vi "Teleop.vi"(10 "Match Info":T1={"Autonomous Elapsed Seconds"=0.0, "TeleOp Elapsed Seconds"=0.0, "Disabled Elapsed Seconds"=0.0, "Visited Autonomous"=FALSE, "Visited TeleOp"=FALSE, "Visited Disabled"=FALSE, "Autonomous Settings"={"Autonomous Style"=enum."Independent", "VI Refnum"=refnum}}, 11 "Call Context":T2) -> ()   [LabVIEW 2017]
doc: "This VI is called for each TeleOp packet received from the DS where the robot is not disabled. It is often used to read from the joysticks and update I/O or to update setpoints for timed control loops. It should complete and return within 20 milliseconds or it may miss DS packets."
uses:
  <vilib>/Rock Robotics/WPI/DriverStation/WPI_DriverStationDerivedRobotMode.ctl
  <vilib>/Rock Robotics/WPI/DriverStation/WPI_DriverStationMatch Info.ctl
  <vilib>/Rock Robotics/WPI/Utilities/WPI_GetSetVariantRefNum.vi
  <vilib>/Rock Robotics/Network Tables/NT Write Boolean Array.vi
  <vilib>/Rock Robotics/Network Tables/NT Write Numeric Array.vi
  <vilib>/Rock Robotics/Network Tables/NT Read Boolean.vi
  <vilib>/Rock Robotics/Network Tables/NT Read Number.vi
panel:
  in  "Lift Select":dbl
  out "Sample Slider 0":dbl(slide) scale=0.0..5.0
  out "Sample Boolean 1":bool
  out "Sample Boolean 0":bool
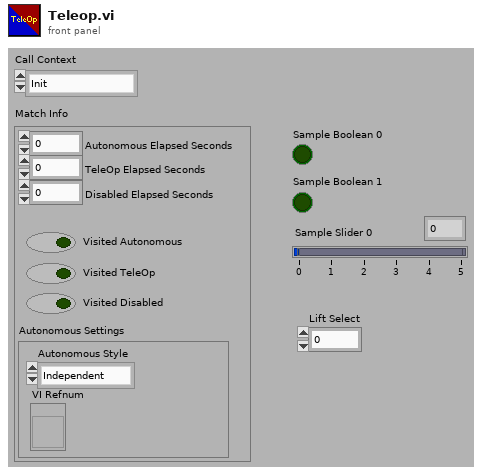
[diagram p1: front panel]
types:
  T1 = typedef "WPI_DriverStationMatch Info.ctl" = cluster{"Autonomous Elapsed Seconds":dbl, "TeleOp Elapsed Seconds":dbl, "Disabled Elapsed Seconds":dbl, "Visited Autonomous":bool, "Visited TeleOp":bool, "Visited Disabled":bool, "Autonomous Settings":cluster{"Autonomous Style":enum16{"Iterative", "Independent"}, "VI Refnum":refnum<vi>}}
  T2 = typedef "WPI_DriverStationDerivedRobotMode.ctl" = enum16{"Init", "Execute", "Stop"}
  T3 = typedef "WPI_JoystickDevRef.ctl" = cluster{"Device":T4}
  T4 = typedef "WPI_JoystickDeviceEnum.ctl" = enum16{"USB 0", "USB 1", "USB 2", "USB 3", "USB 4", "USB 5"}
  T5 = typedef "WPI_MotorControlDeviceRef.ctl" = cluster{"DeviceStatus":errorcluster, "Type":T6, "PWM":cluster{"PWM Channel":T7, "DeadBand":T8}, "CAN":cluster{"Device Number":u8, "SetOutput VI Ref":variant, "GetOutput VI Ref":variant, "Enable VI Ref":variant, "Disable VI Ref":variant, "Data":variant}, "Invert":bool, "DIO PWM":cluster{"PWM \"Enable\" Channel":T7, "DIOChannel":T9, "PWM Rate":dbl}}
  T6 = typedef "WPI_MotorControlType.ctl" = enum16{"PWM", "CAN", "DIO PWM"}
  T7 = typedef "FPGA_DIOPWMChannel.ctl" = enum8{"PWM 0", "PWM 1", "PWM 2", "PWM 3", "PWM 4", "PWM 5", "PWM 6", "PWM 7", "PWM 8", "PWM 9", "PWM MXP 0", "PWM MXP 1", "PWM MXP 2", "PWM MXP 3", "PWM MXP 4", "PWM MXP 5", "PWM MXP 6", "PWM MXP 7", "PWM MXP 8", "PWM MXP 9", "Invalid"}
  T8 = typedef "WPI_PWMDeadband.ctl" = cluster{"Name":string, "maxPositivePwm":i32, "minPositivePwm":i32, "centerPwm":i32, "maxNegativePwm":i32, "minNegativePwm":i32, "angularRange":u16}
  T9 = typedef "FPGA_DIOChannel.ctl" = enum8{"DIO 0", "DIO 1", "DIO 2", "DIO 3", "DIO 4", "DIO 5", "DIO 6", "DIO 7", "DIO 8", "DIO 9", "DIO MXP 0", "DIO MXP 1", "DIO MXP 2", "DIO MXP 3", "DIO MXP 4", "DIO MXP 5", "DIO MXP 6", "DIO MXP 7", "DIO MXP 8", "DIO MXP 9", "DIO MXP 10", "DIO MXP 11", "DIO MXP 12", "DIO MXP 13", "DIO MXP 14", "DIO MXP 15", "SPI Port CS1", "SPI Port CS2", "SPI Port CS3", "SPI Port MISO", "SPI Port MOSI", "Invalid"}
  T10 = typedef "WPI_RobotDriveDevRef.ctl" = cluster{"DevStatus":errorcluster, "Motors[]":T5[], "Square Inputs":bool, "Max Output":dbl}
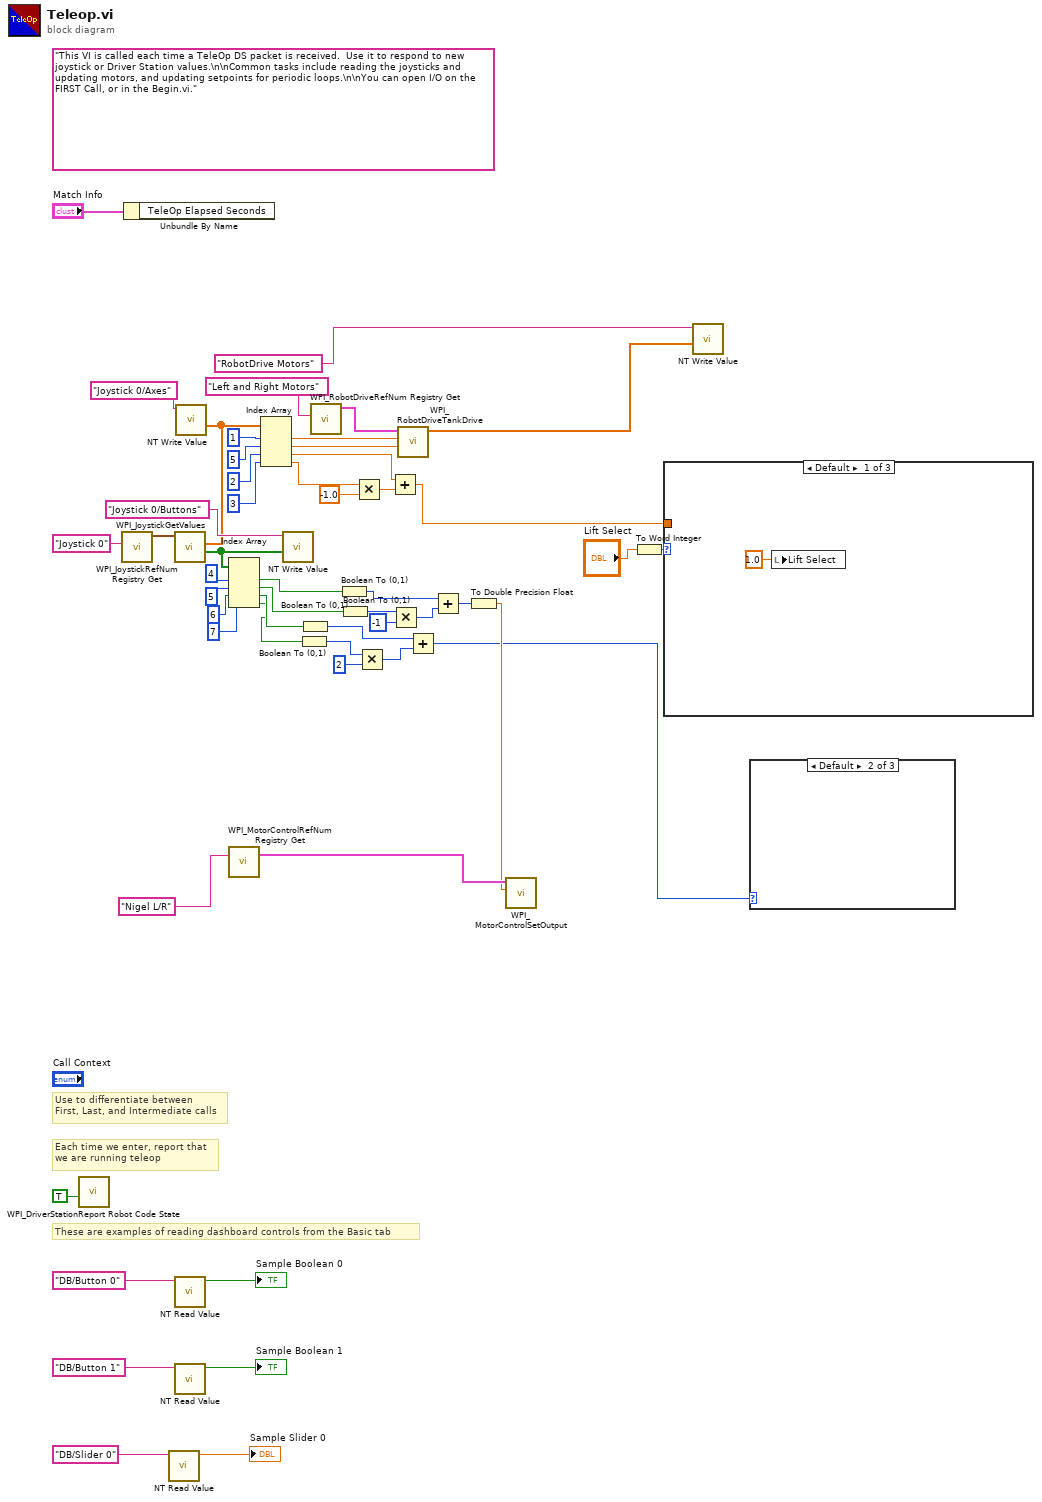
[diagram p0: block diagram]
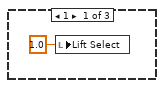
[diagram p2: hidden frame]
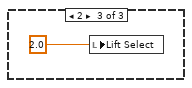
[diagram p3: hidden frame]
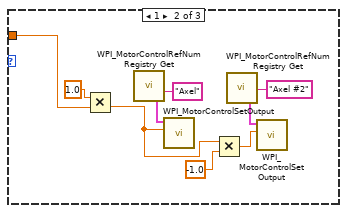
[diagram p4: hidden frame]
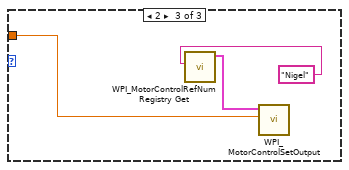
[diagram p5: hidden frame]
diagram:
  (unwired) "This VI is called each time a TeleOp DS packet is received.  Use it to respond to new joystick or Driver Station values.\n\nCommon tasks include reading the joysticks and updating motors, and updating setpoints for periodic loops.\n\nYou can open I/O on the FIRST Call, or in the Begin.vi."
  # "These are examples of reading dashboard controls from the Basic tab"
  # "Each time we enter, report that\nwe are running teleop"
  # "Use to differentiate between\nFirst, Last, and Intermediate calls"
  n1 = call <vilib>:"WPI_DriverStationReport Robot Code State.vi"("TeleOp"=TRUE ("Autonomous")) -> ()  [unwired: 10 in, 1 out]
  n2 = call <vilib>:"WPI_JoystickRefNum Registry Get.vi"("refnum name"="Joystick 0") -> ("JoystickDevRef"=w48:T3)  [unwired: 1 in, 9 out]
  n3 = Unbundle By Name("Match Info") -> ()  [unwired: 1 out]
  n4 = call-poly <vilib>:"NT Read Value.vi"("Name"="DB/Slider 0" ("refnum name")) -> ("Numeric"=→"Sample Slider 0":dbl)  [unwired: 9 in, 1 out]
  n5 = call <vilib>:"WPI_JoystickGetValues.vi"("JoystickDevRef"=w48) -> ("Buttons"=w27:bool[], "Axes"=w43:dbl[])  [unwired: 6 in, 3 out]
  n6 = call-poly <vilib>:"NT Read Value.vi"("Name"="DB/Button 0" ("refnum name")) -> ("Boolean"=→"Sample Boolean 0":bool)  [unwired: 9 in, 1 out]
  n7 = call-poly <vilib>:"NT Read Value.vi"("Name"="DB/Button 1" ("refnum name")) -> ("Boolean"=→"Sample Boolean 1":bool)  [unwired: 9 in, 1 out]
  n8 = call-poly <vilib>:"NT Write Value.vi"("Numeric Array"=w43, "Name"="Joystick 0/Axes") -> ()  [unwired: 9 in, 1 out]
  n9 = Index Array(array=w27, index #1=4 ("index"), index #2=5 ("index"), index #3=6 ("index"), index #4=7 ("index")) -> (element #1=w21:bool, element #2=w20:bool, element #3=w12:bool, element #4=w11:bool)
  n10 = call <vilib>:"WPI_MotorControlRefNum Registry Get.vi"("refnum name"="Nigel L/R") -> ("MotorControlDevRef"=w5:T5)  [unwired: 9 in, 1 out]
  n11 = Index Array(array=w43, index #1=1 ("index"), index #2=5 ("index"), index #3=2 ("index"), index #4=3 ("index")) -> (element #1=w28:dbl, element #2=w46:dbl, element #3=w23:dbl, element #4=w26:dbl)
  n12 = call-poly <vilib>:"NT Write Value.vi"("Boolean Array"=w27, "Name"="Joystick 0/Buttons") -> ()  [unwired: 9 in, 1 out]
  n13 = Boolean To (0,1)(Boolean=w11) -> (0, 1=w10:i16)
  n14 = Boolean To (0,1)(Boolean=w12) -> (0, 1=w8:i16)
  n15 = call <vilib>:"WPI_RobotDriveRefNum Registry Get.vi"("refnum name"="Left and Right Motors") -> ("RobotDriveDevRef"=w50:T10)  [unwired: 1 in, 9 out]
  n16 = Boolean To (0,1)(Boolean=w21) -> (0, 1=w18:i16)
  n17 = Boolean To (0,1)(Boolean=w20) -> (0, 1=w19:i16)
  n18 = Multiply(x=w26, y=-1.0) -> (x*y=w22:dbl)
  n19 = Multiply(x=w10, y=i16 2) -> (x*y=w7:i16)
  n20 = Add(x=w23, y=w22) -> (x+y=w6:dbl)
  n21 = Multiply(x=w19, y=i16 -1) -> (x*y=w17:i16)
  n22 = call <vilib>:"WPI_RobotDriveTankDrive.vi"("Right axis value"=w46, "Left axis value"=w28, "RobotDriveDevRef"=w50) -> ("Motor Values"=w36:dbl[])  [unwired: 6 in, 2 out]
  n23 = Add(x=w8, y=w7) -> (x+y=w1:i16)
  n24 = Add(x=w18, y=w17) -> (x+y=w15:i16)
  n25 = To Double Precision Float(number=w15) -> (double precision float=w4:dbl)
  n26 = call <vilib>:"WPI_MotorControlSetOutput.vi"("Output"=w4, "MotorControlDevRef"=w5) -> ()  [unwired: 7 in, 3 out]
  n27 = To Word Integer(number="Lift Select") -> (16bit integer=w2:i16)
  n28 = case shown="Default" w2 {
    tunnel: w6 -> [_ w56 w65]
    frame Default {
      n29 = local write "Lift Select"(1.0 ("Lift Select")) -> ()
    }
    frame 1 {
      n30 = Multiply(x=1.0, y=w56) -> (x*y=w55:dbl)
      n31 = call <vilib>:"WPI_MotorControlRefNum Registry Get.vi"("refnum name"="Axel") -> ("MotorControlDevRef"=w61:T5)  [unwired: 9 in, 1 out]
      n32 = call <vilib>:"WPI_MotorControlSetOutput.vi"("Output"=w55, "MotorControlDevRef"=w61) -> ()  [unwired: 7 in, 3 out]
      n33 = Multiply(x=w55, y=-1.0) -> (x*y=w57:dbl)
      n34 = call <vilib>:"WPI_MotorControlRefNum Registry Get.vi"("refnum name"="Axel #2") -> ("MotorControlDevRef"=w60:T5)  [unwired: 9 in, 1 out]
      n35 = call <vilib>:"WPI_MotorControlSetOutput.vi"("Output"=w57, "MotorControlDevRef"=w60) -> ()  [unwired: 7 in, 3 out]
    }
    frame 2 {
      n36 = call <vilib>:"WPI_MotorControlRefNum Registry Get.vi"("refnum name"="Nigel") -> ("MotorControlDevRef"=w64:T5)  [unwired: 9 in, 1 out]
      n37 = call <vilib>:"WPI_MotorControlSetOutput.vi"("Output"=w65, "MotorControlDevRef"=w64) -> ()  [unwired: 7 in, 3 out]
    }
  }
  n38 = call-poly <vilib>:"NT Write Value.vi"("Numeric Array"=w36, "Name"="RobotDrive Motors") -> ()  [unwired: 9 in, 1 out]
  n39 = case shown="Default" w1 {
    frame 1 {
      n40 = local write "Lift Select"(1.0 ("Lift Select")) -> ()
    }
    frame Default {
    }
    frame 2 {
      n41 = local write "Lift Select"(2.0 ("Lift Select")) -> ()
    }
  }
